vi "LJM logger get working directory.vi"(10 "Application Name":string="LJlogger") -> (0 "Error":bool, 3 "Working Directory":path)   [LabVIEW 2026]
uses:
  <vilib>/registry/registry.llb/Registry RtKey.ctl
  <vilib>/registry/registry.llb/Read Registry Value Simple STR.vi
  <vilib>/registry/registry.llb/Write Registry Value Simple STR.vi
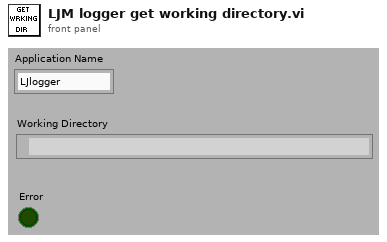
[diagram p1: front panel]
types:
  T1 = typedef "Registry RtKey.ctl" = enum32{"HKEY_CLASSES_ROOT", "HKEY_CURRENT_USER", "HKEY_LOCAL_MACHINE", "HKEY_USERS", "HKEY_PERFORMANCE_DATA", "HKEY_CURRENT_CONFIG", "HKEY_DYN_DATA"}
  T2 = enum16{"open", "open or create", "create or replace", "create", "open (read only)"}
  T3 = typedef "Registry refnum.ctl" = refnum<k1>
  T4 = enum32{"existing file", "new file", "new or existing file", "existing dir", "new dir", "new or existing dir", "existing file (use LLBs)", "new file (use LLBs)", "new or existing file (use LLBs)", "new or existing file or directory (use LLBs)"}
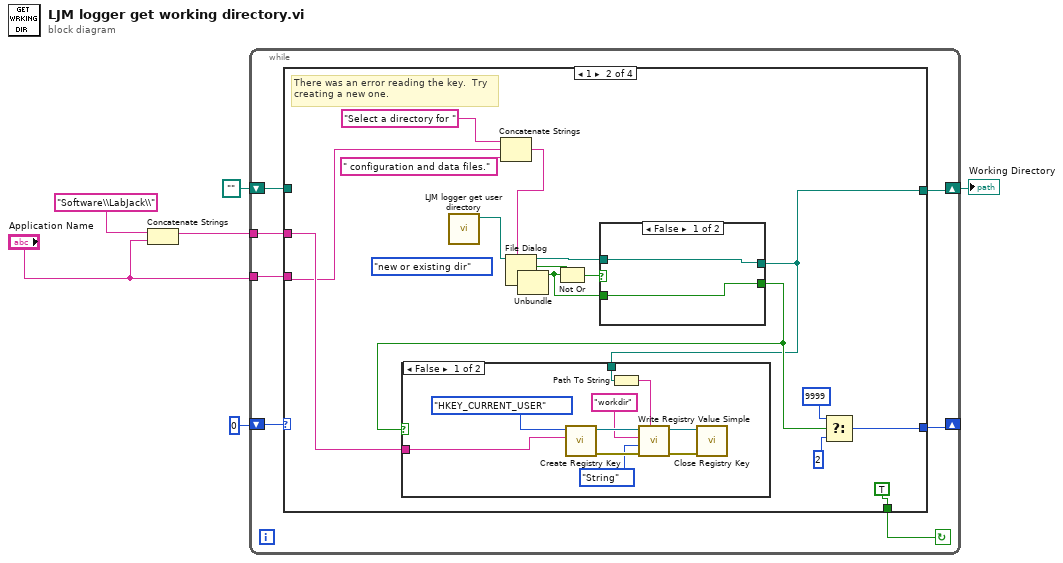
[diagram p0: block diagram]
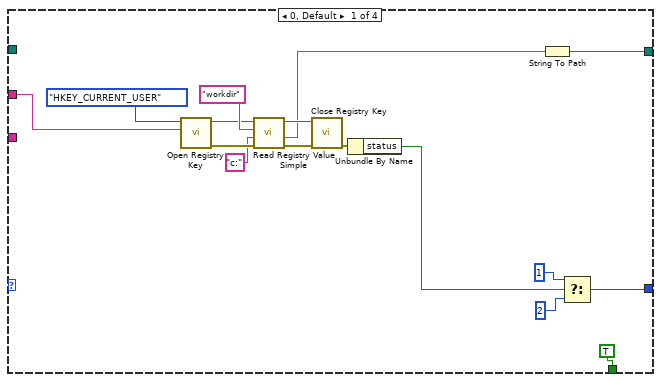
[diagram p2: hidden frame]
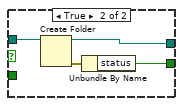
[diagram p4: hidden frame]
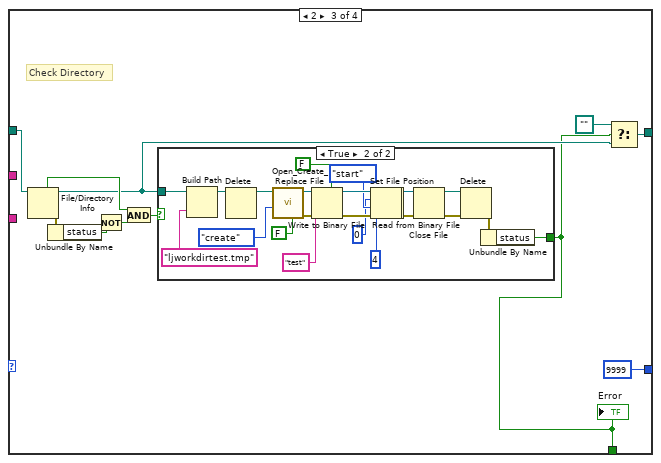
[diagram p5: hidden frame]
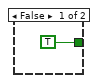
[diagram p6: hidden frame]
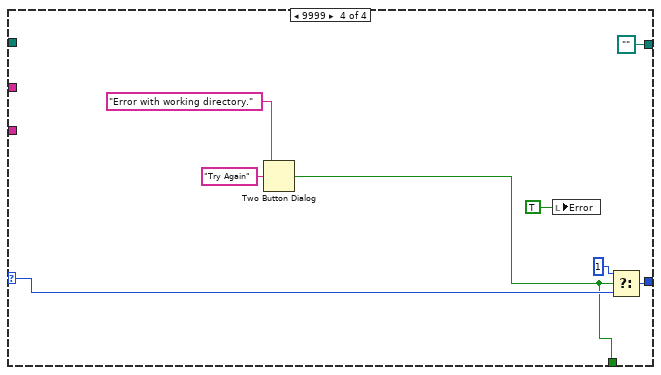
[diagram p7: hidden frame]
diagram:
  n1 = Concatenate Strings("Software\\LabJack\\" ("subkey"), "Application Name") -> (w1:string)
  n2 = while {
    tunnel: w1 -> [w7]
    tunnel: "Application Name" -> [w8]
    shift-left: path "" -> [w9]
    shift-right: [w11] -> w4
    shift-left: 0 -> [w13]
    shift-right: [w12] -> _
    stop <- w10 continue-if-true
    n3 = case shown="1" w13 {
      selector: w13 -> [_ _ _ w102]
      tunnel: [w20 w42 9999 w103] -> w12
      tunnel: [w18 w37 w64 path "" ("dup directory path")] -> w11
      tunnel: [TRUE TRUE w66 w100] -> w10
      tunnel: w9 -> [_ _ w73 _]
      tunnel: w8 -> [_ w33 _ _]
      tunnel: w7 -> [w14 w36 _ _]
      frame 0, Default {
        n4 = call <vilib>:"Open Registry Key.vi"("subkey"=w14, "root key (HKEY_LOCAL_MACHINE)"=Registry_RtKey."HKEY_CURRENT_USER") -> ("error out"=w28:errorcluster, "refnum out"=w25:T3)  [unwired: 8 in]
        n5 = call-poly <vilib>:"Read Registry Value Simple.vi"("error in (no error)"=w28, "default data"="c:", "value"="workdir", "refnum"=w25) -> ("error out"=w23:errorcluster, "String/Binary data"=w19:string, "refnum out"=w24:T3)  [unwired: 2 in, 1 out]
        n6 = call <vilib>:"Close Registry Key.vi"("error in (no error)"=w23, "refnum"=w24) -> ("error out"=w22:errorcluster)  [unwired: 5 in]
        n7 = Unbundle By Name(w22) -> ("status"=w21:bool)
        n8 = String To Path(string=w19) -> (path=w18:path)
        n9 = Select(t=1, s=w21, f=2) -> (s? t:f=w20:i32)
      }
      frame 1 {
        (unwired) T4."new or existing dir" ("select mode (2)")
        # "There was an error reading the key.  Try\ncreating a new one."
        n10 = call "LJM logger get user directory.vi"() -> ("User Directory"=w31:path)  [unwired: 11 in]
        n11 = Concatenate Strings("Select a directory for " ("prompt"), w33, " configuration and data files." ("Substring")) -> (w32:string)
        n12 = File Dialog(7:w32, 11:w31) -> (0:w30:errorcluster, 1:w43:bool, 2:w45:bool, 3:w46:path)  [unwired: 5 in]
        n13 = Unbundle(w30) -> ()  [unwired: 3 out]
        n14 = Not Or(1:w43, 2:w45) -> (0:w44:bool)
        n15 = case shown="False" w44 {
          tunnel: w46 -> [w57 w62]
          tunnel: [w57 w60] -> w37
          tunnel: [w58 w59] -> w38
          tunnel: w43 -> [w58 _]
          frame False {
          }
          frame True {
            n16 = Create Folder(path (use dialog)=w62) -> (created path=w60:path, error out=w61:errorcluster)  [unwired: 2 in, 1 out]
            n17 = Unbundle By Name(w61) -> ("status"=w59:bool)
          }
        }
        n18 = case shown="False" w38 {
          tunnel: w37 -> [w49 _]
          tunnel: w36 -> [w47 _]
          frame False {
            n19 = call <vilib>:"Create Registry Key.vi"("subkey"=w47, "root key (HKEY_LOCAL_MACHINE)"=Registry_RtKey."HKEY_CURRENT_USER") -> ("error out"=w55:errorcluster, "refnum out"=w54:T3)  [unwired: 7 in, 1 out]
            n20 = Path To String(path=w49) -> (string=w48:string)
            n21 = call-poly <vilib>:"Write Registry Value Simple.vi"("String/Binary data"=w48, "error in (no error)"=w55, "simple data type"=enum16{"String", "Binary", "DWORD"}."String", "value"="workdir", "refnum"=w54) -> ("error out"=w52:errorcluster, "refnum out"=w53:T3)  [unwired: 3 in]
            n22 = call <vilib>:"Close Registry Key.vi"("error in (no error)"=w52, "refnum"=w53) -> ()  [unwired: 5 in, 1 out]
          }
          frame True {
          }
        }
        n23 = Select(t=9999, s=w38, f=2) -> (s? t:f=w42:i32)
      }
      frame 2 {
        # "Check Directory"
        n24 = File/Directory Info(path=w73) -> (path out=w67:path, directory=w69:bool, error out=w72:errorcluster)  [unwired: 1 in, 4 out]
        n25 = Unbundle By Name(w72) -> ("status"=w71:bool)
        n26 = Not(x=w71) -> (.not. x?=w70:bool)
        n27 = And(x=w69, y=w70) -> (x .and. y?=w68:bool)
        n28 = case shown="True" w68 {
          tunnel: w67 -> [_ w90]
          tunnel: [TRUE ("status") w82] -> w66
          frame False {
          }
          frame True {
            n29 = Build Path(base path=w90, name or relative path="ljworkdirtest.tmp") -> (appended path=w88:path)
            n30 = Delete(path (use dialog)=w88) -> (deleted path=w97:path)  [unwired: 4 in, 2 out]
            n31 = call <vilib>:"Open_Create_Replace File.vi"("advisory dialog? (display:T)"=FALSE, "function (open:0)"=T2."create", "file path"=w97) -> ("error out"=w93:errorcluster, "refnum"=w96:refnum<file>)  [unwired: 5 in, 2 out]
            n32 = Write to Binary File(file (use dialog)=w96, data="test", error in=w93, 5:FALSE ("prepend array or string size? (T)")) -> (refnum out=w95:refnum<file>, error out=w92:errorcluster)  [unwired: 2 in, 1 out]
            n33 = Set File Position(offset (in bytes) (0)=0 ("pos offset (0)"), refnum=w95, from (0:start)=enum16{"start", "end", "current"}."start" ("pos mode (0:2)"), error in=w92) -> (refnum out=w76:refnum<file>, error out=w75:errorcluster)
            n34 = Read from Binary File(8:w75, 10:4 ("count"), 11:w76) -> (0:w91:errorcluster, 3:w94:refnum<file>)  [unwired: 3 in, 2 out]
            n35 = Close File(refnum=w94, error in=w91) -> (path=w85:path, error out=w84:errorcluster)
            n36 = Delete(path (use dialog)=w85, error in=w84) -> (error out=w83:errorcluster)  [unwired: 3 in, 2 out]
            n37 = Unbundle By Name(w83) -> ("status"=w82:bool)
          }
        }
        "Error" <- w66
        n38 = Select(t=path "", s=w66, f=w67) -> (s? t:f=w64:path)
      }
      frame 9999 {
        n39 = Two Button Dialog(message="Error with working directory.", 2:"Try Again" ("T button name (\"OK\")")) -> (T button?=w100:bool)  [unwired: 1 in]
        n40 = local write "Error"(TRUE ("Error")) -> ()
        n41 = Select(t=1, s=w100, f=w102) -> (s? t:f=w103:i32)
      }
    }
  }
  "Working Directory" <- w4
